vi "Verify Configuration.vi"(0 "eye scan in":refnum<class "niHighSpeedSerial N Point Eye Scan v1 Host.lvclass">, 11 "error in":errorcluster) -> (4 "eye scan out":refnum<class "niHighSpeedSerial N Point Eye Scan v1 Host.lvclass">, 15 "error out":errorcluster)   [LabVIEW 2014, in "niHighSpeedSerial N Point Eye Scan v1 Host.lvclass"]
doc: "Validates that the current configuration is valid before starting Eye Scan on the FPGA.\n\n<B>Input Parameters</B>\n\n<B>eye scan in</B> Takes in a reference to your session from the previous VI.\n\n<B>error in</B> describes error conditions that occur before this node runs. This input provides standard 'error in' functionality.\n\n<B>Output Parameters</B>\n\n<B>eye scan out</B> passes a reference to your session to the next VI.\n\n<B>error out</B> contains error information. This output provides standard 'error out' functionality."
uses:
  <instrlib>/niHighSpeedSerial/Eye Scan/v1/Host/Impl/N Point Eye Scan/niHighSpeedSerial N Point Eye Scan v1 Host.lvclass
  <instrlib>/niHighSpeedSerial/Eye Scan/v1/Host/Impl/N Point Eye Scan/niHighSpeedSerial N Point Eye Scan v1 Host.lvclass/niHighSpeedSerial N Point Eye Scan v1 Host.ctl
  <vilib>/Utility/error.llb/Error Cluster From Error Code.vi
  <instrlib>/niHighSpeedSerial/Eye Scan/v1/Host/Eye Scan/niHighSpeedSerial Eye Scan v1 Host.lvclass
  <vilib>/ErrorRing/Error Ring.xnode
  <instrlib>/niHighSpeedSerial/Eye Scan/v1/Host/Common/niHighSpeedSerial Eye Scan Common v1 Host.lvlib
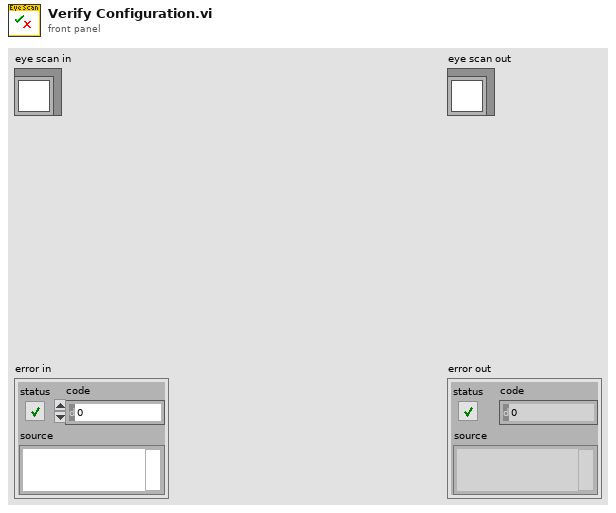
[diagram p1: front panel]
types:
  T1 = typedef "N Point Eye Scan v1 Host.lvclass/Private Data.ctl" = cluster{"array of points to measure":T2[], "n point eye scan point iterator":refnum<class "niHighSpeedSerial N Point Eye Scan Point Iterator v1 Host.lvclass">}
  T2 = typedef "niHighSpeedSerial Eye Scan Common v1 Host.lvlib/Point Offsets.ctl" = cluster{"horizontal offset":i16, "vertical offset":i8}
  T3 = typedef "niHighSpeedSerial Eye Scan Common v1 Host.lvlib/RX Output Divider.ctl" = enum16{"1", "2", "4", "8", "16"}
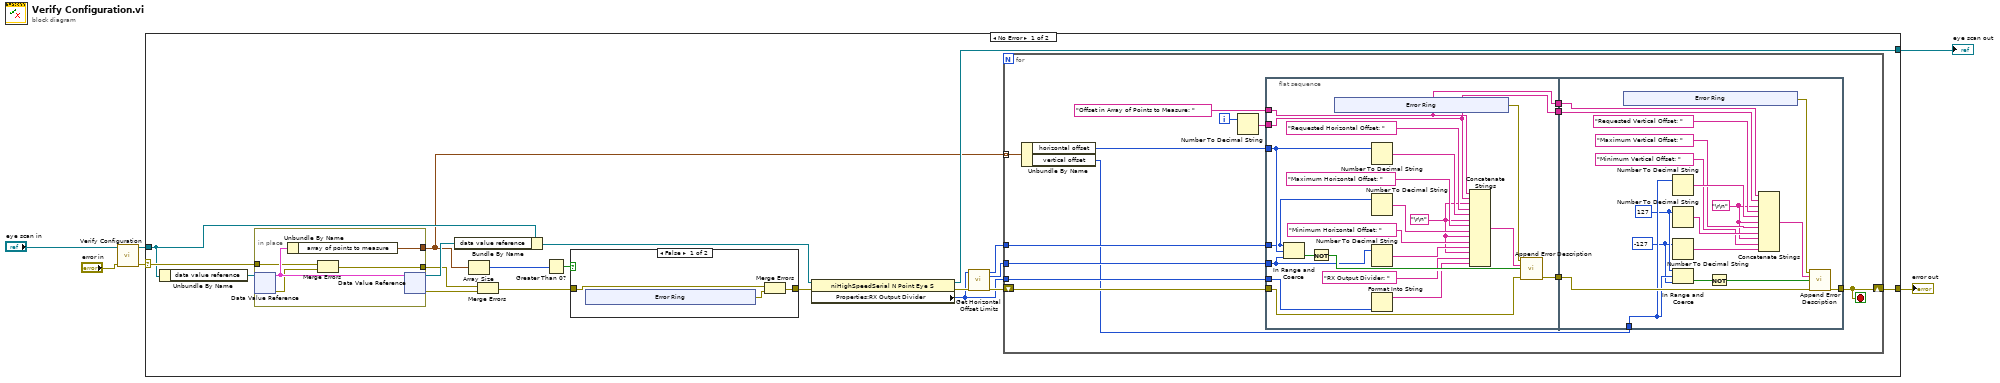
[diagram p0: block diagram]
diagram:
  n1 = call-parent "Verify Configuration.vi"("eye scan in"="eye scan in", "error in"="error in") -> ("eye scan out"=w2:refnum<class "niHighSpeedSerial N Point Eye Scan v1 Host.lvclass">, "error out"=w1:errorcluster)  [unwired: 12 in]
  n2 = case shown="No Error" w1 {
    selector: w1 -> [w18 w100]
    tunnel: w2 -> [w16 w101]
    tunnel: [w13 w101] -> w6
    tunnel: [w21 w100] -> w5
    frame No Error {
      n3 = Unbundle By Name(w16) -> ("data value reference"=w25:refnum<data-value>)
      n4 = in-place {
        in-place-border: [w99] -> w12
        in-place-border: w18 -> [w97]
        in-place-border: [w95] -> w23
        n5 = in-place-dvr #1(w25) -> (w98:T1, w96:errorcluster)
        n6 = Unbundle By Name(w98) -> ("array of points to measure"=w99:T2[])
        n7 = Merge Errors(w97, w96) -> (w95:errorcluster)
        n8 = in-place-dvr #1(w98) -> (w24:refnum<data-value>, w22:errorcluster)
      }
      n9 = Bundle By Name(cluster=w16, "data value reference"=w24) -> (w15:refnum<class "niHighSpeedSerial N Point Eye Scan v1 Host.lvclass">)
      n10 = Array Size(array=w12) -> (size(s)=w11:i32)
      n11 = Merge Errors(w23, w22) -> (w8:errorcluster)
      n12 = Greater Than 0?(x=w11) -> (x > 0?=w10:bool)
      n13 = case shown="False" w10 {
        tunnel: [w28 w33] -> w9
        tunnel: w8 -> [w27 w33]
        frame False {
          n14 = xnode "Error Ring"() -> ("error out"=w26:errorcluster)
          n15 = Merge Errors(w27, w26) -> (w28:errorcluster)
        }
        frame True {
        }
      }
      n16 = property class="niHighSpeedSerial N Point Eye S"(reference=w15, error in=w9) -> (reference out=w13:refnum<class "niHighSpeedSerial N Point Eye Scan v1 Host.lvclass">, error out=w14:errorcluster, "Properties:RX Output Divider"=w7:T3)
      n17 = call <instrlib>:"Get Horizontal Offset Limits.vi"("rx output divider"=w7, "error in"=w14) -> ("maximum"=w20:i16, "minimum"=w19:i16, "error out"=w17:errorcluster)  [unwired: 10 in, 1 out]
      n18 = for {
        tunnel: w12 -> [w47] mode=indexing
        shift-right: [w37] -> w21
        shift-left: w17 -> [w45]
        tunnel: w20 -> [w43]
        tunnel: w19 -> [w42]
        tunnel: w7 -> [w41]
        i -> [w46]
        stop <- w37 stop-if-true
        n19 = Unbundle By Name(w47) -> ("horizontal offset"=w44:i16, "vertical offset"=w36:i8)
        n20 = Number To Decimal String(number=w46) -> (decimal integer string=w39:string)  [unwired: 1 in]
        n21 = flat-sequence {
          tunnel: w45 -> [w64]
          tunnel: w44 -> [w62]
          tunnel: w43 -> [w59]
          tunnel: w42 -> [w56]
          tunnel: w41 -> [w52]
          tunnel: "Offset in Array of Points to Measure: " ("append string (\"\")") -> [w49]
          tunnel: w39 -> [w48]
          tunnel: [w50] -> w38
          tunnel: [w49] -> w35
          tunnel: [w48] -> w34
          tunnel: w38 -> [w89]
          tunnel: [w88] -> w37
          tunnel: w36 -> [w85]
          tunnel: w35 -> [w84]
          tunnel: w34 -> [w83]
          frame #0 {
            w54 = "\r\n"
            n22 = In Range and Coerce(upper limit=w59, x=w62, lower limit=w56) -> (In Range?=w68:bool)  [unwired: 1 out]
            n23 = Not(x=w68) -> (.not. x?=w66:bool)
            n24 = xnode "Error Ring"() -> ("error out"=w67:errorcluster)
            n25 = Number To Decimal String(number=w62) -> (decimal integer string=w61:string)  [unwired: 1 in]
            n26 = Number To Decimal String(number=w59) -> (decimal integer string=w58:string)  [unwired: 1 in]
            n27 = Number To Decimal String(number=w56) -> (decimal integer string=w55:string)  [unwired: 1 in]
            n28 = Format Into String(w52) -> (resulting string=w51:string)  [unwired: 3 in, 1 out]
            n29 = Concatenate Strings(w49, w48, w54, "Requested Horizontal Offset: " ("string"), w61, w54, "Maximum Horizontal Offset: " ("string"), w58, w54, "Minimum Horizontal Offset: " ("string"), w55, w54, "RX Output Divider: " ("string"), w51) -> (w65:string)
            n30 = call <instrlib>:"Append Error Description.vi"("error to append"=w67, "append string (\"\")"=w65, "generate error?"=w66, "error in"=w64) -> ("error out"=w50:errorcluster)  [unwired: 11 in]
          }
          frame #1 {
            w74 = i8 -127 ("lower limit")
            w79 = i8 127 ("upper limit")
            w77 = "\r\n"
            n31 = xnode "Error Ring"() -> ("error out"=w90:errorcluster)
            n32 = Number To Decimal String(number=w85) -> (decimal integer string=w81:string)  [unwired: 1 in]
            n33 = Number To Decimal String(number=w79) -> (decimal integer string=w78:string)  [unwired: 1 in]
            n34 = Number To Decimal String(number=w74) -> (decimal integer string=w75:string)  [unwired: 1 in]
            n35 = In Range and Coerce(upper limit=w79, x=w85, lower limit=w74) -> (In Range?=w87:bool)  [unwired: 1 out]
            n36 = Not(x=w87) -> (.not. x?=w86:bool)
            n37 = Concatenate Strings(w84, w83, w77, "Requested Vertical Offset: " ("string"), w81, w77, "Maximum Vertical Offset: " ("string"), w78, w77, "Minimum Vertical Offset: " ("string"), w75) -> (w73:string)
            n38 = call <instrlib>:"Append Error Description.vi"("error to append"=w90, "append string (\"\")"=w73, "generate error?"=w86, "error in"=w89) -> ("error out"=w88:errorcluster)  [unwired: 11 in]
          }
        }
      }
    }
    frame Error {
    }
  }
  "error out" <- w5
  "eye scan out" <- w6
